vi "PegaRetaOrientacaoOuPosicao.vi"(4 "Goal Width":u32, 5 "Field Length":u32, 6 "Orientação inimigo":dbl format="%#_13g", 7 "Meio?":bool=TRUE, 8 "Y bola":dbl format="%#_13g", 9 "X bola":dbl format="%#_13g", 10 "Y inimigo":dbl format="%#_13g", 11 "X inimigo":dbl format="%#_13g") -> (0 "Orientação goleiro":dbl format="%#_13g", 2 "Y goleiro":dbl format="%#_13g", 3 "X goleiro":dbl format="%#_13g")   [LabVIEW 2017]
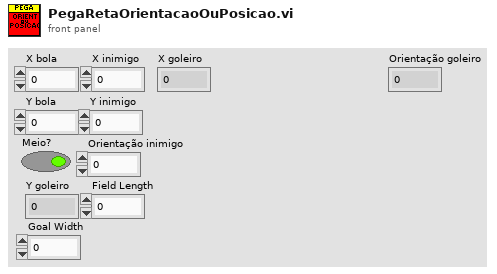
[diagram p1: front panel]
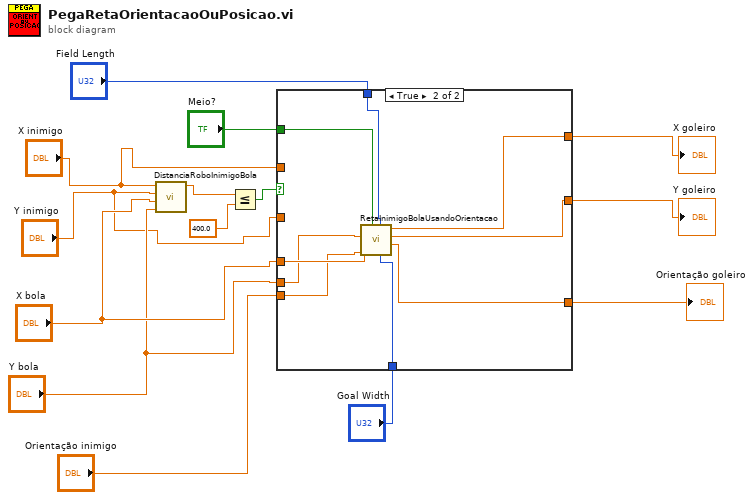
[diagram p0: block diagram]
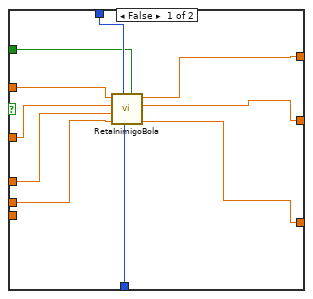
[diagram p2: hidden frame]
diagram:
  n1 = call "DistanciaRoboInimigoBola.vi"("Y bola"="Y bola", "X bola"="X bola", "Y inimigo"="Y inimigo", "X inimigo"="X inimigo") -> ("Distância"=w14:dbl)  [unwired: 5 in, 2 out]
  n2 = Less Or Equal?(x=w14, y=400.0) -> (x <= y?=w12:bool)
  n3 = case shown="True" w12 {
    tunnel: "X bola" -> [w24 w33]
    tunnel: "Y bola" -> [w23 w32]
    tunnel: "Orientação inimigo" -> [_ w31]
    tunnel: "Meio?" -> [w15 w30]
    tunnel: "Goal Width" -> [w19 w29]
    tunnel: "Field Length" -> [w20 w28]
    tunnel: [w18 w27] -> w5
    tunnel: [w17 w26] -> w4
    tunnel: [w16 w25] -> w3
    tunnel: "X inimigo" -> [w22 _]
    tunnel: "Y inimigo" -> [w21 _]
    frame False {
      n4 = call "RetaInimigoBola.vi"("Meio?"=w15, "Goal width"=w19, "Field lenght"=w20, "Y bola"=w23, "X bola"=w24, "Y inimigo"=w21, "X inimigo"=w22) -> ("Orientação"=w16:dbl, "Y goleiro"=w17:dbl, "X goleiro"=w18:dbl)  [unwired: 2 in]
    }
    frame True {
      n5 = call "RetaInimigoBolaUsandoOrientacao.vi"("Goal Width"=w29, "Field length"=w28, "Meio?"=w30, "Orientação inimigo"=w31, "Y bola"=w32, "X bola"=w33) -> ("Orientação goleiro"=w25:dbl, "Y golerio"=w26:dbl, "X goleiro"=w27:dbl)  [unwired: 3 in]
    }
  }
  "X goleiro" <- w5
  "Y goleiro" <- w4
  "Orientação goleiro" <- w3
